vi "Convex Hull 2D (GiftWrap).vi"(0 "Points":sgl[][](array[numeric])=[[0.0, 0.0, 0.0], [10.0, 0.0, 0.0], [10.0, 10.0, 0.0], [0.0, 10.0, 0.0], [50.0, 50.0, 0.0], [60.0, 50.0, 0.0], [60.0, 60.0, 0.0], [50.0, 60.0, 0.0]]) -> (1 "Convex Hull lines":T1[](array[typedef]), 2 "Convex Hull vertices":sgl[][](array[numeric]))   [LabVIEW 2016]
uses:
  Typedefs/Edge, indexed.ctl
  Subroutines/Cross product 3D.vi
  Subroutines/Unit vector.vi
panel:
  # "PN 17/03/2015"
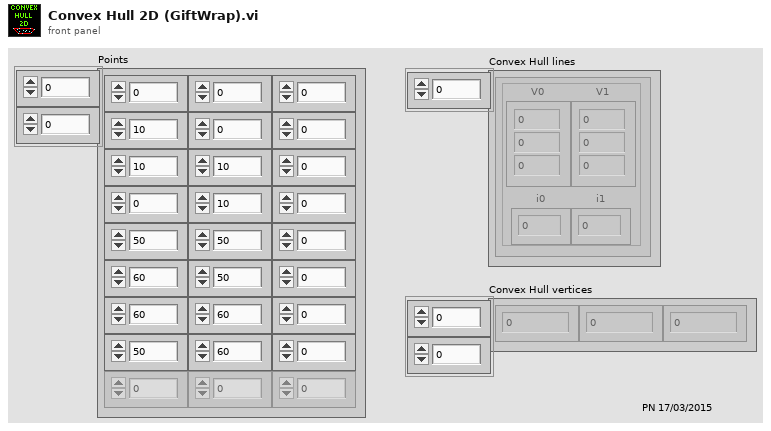
[diagram p1: front panel]
types:
  T1 = typedef "Edge, indexed.ctl" = cluster{"V0":sgl[], "V1":sgl[], "i0":i32, "i1":i32}
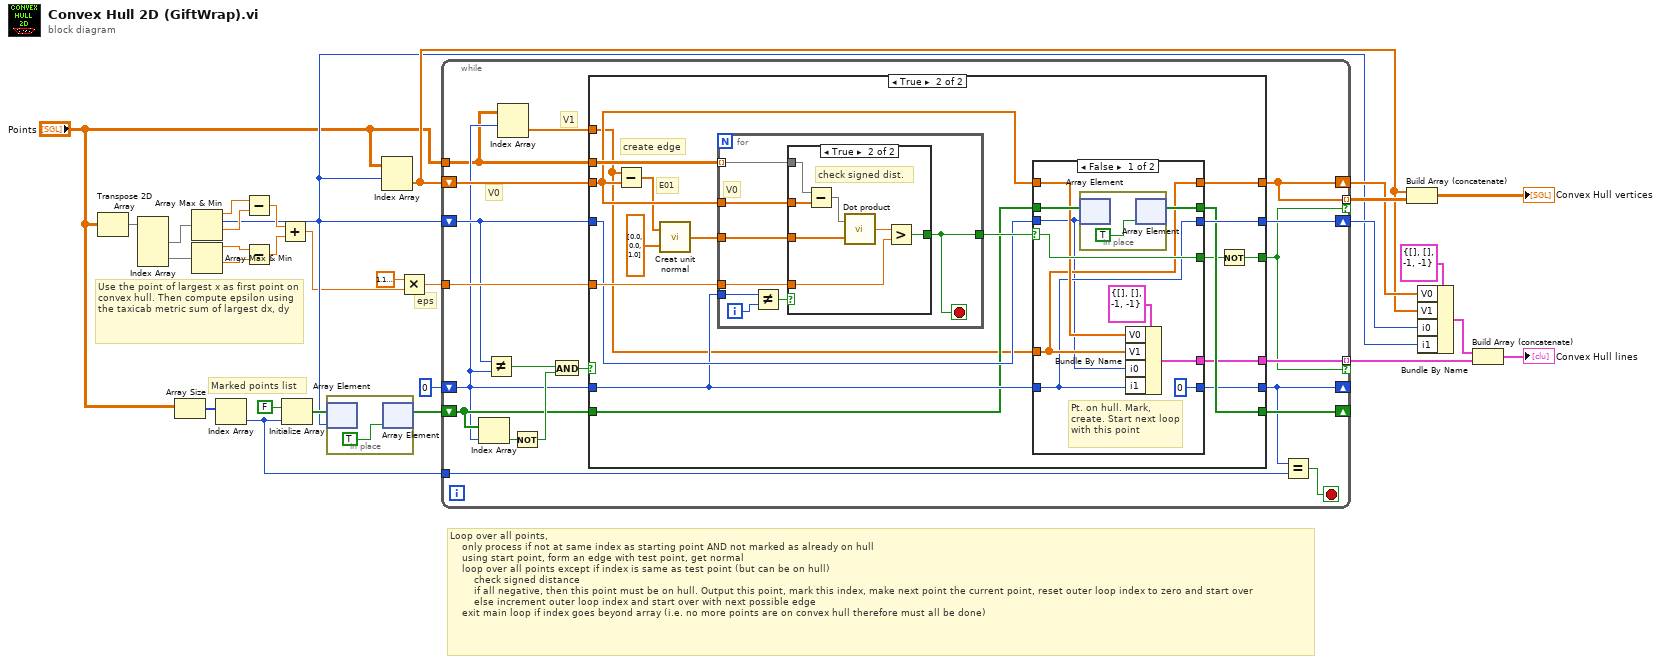
[diagram p0: block diagram]
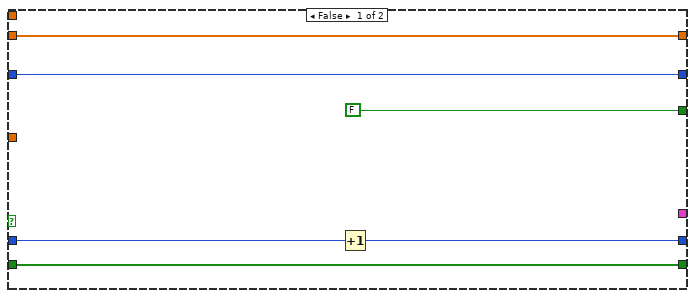
[diagram p2: hidden frame]
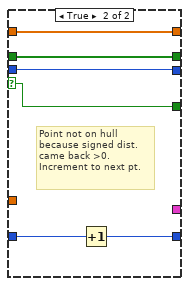
[diagram p3: hidden frame]
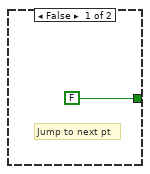
[diagram p4: hidden frame]
diagram:
  # "Use the point of largest x as first point on convex hull. Then compute epsilon using the taxicab metric sum of largest dx, dy"
  # "Loop over all points,\n    only process if not at same index as starting point AND not marked as already on hull\n    using start point, form an edge with test point, get normal\n    loop over all points except if index is same as test point (but can be on hull)\n        check signed distance\n        if all negative, then this point must be on hull. Output this point, mark this index, make next point the current point, reset outer loop index to zero and start over\n        else increment outer loop index and start over with next possible edge\n    exit main loop if index goes beyond array (i.e. no more points are on convex hull therefore must all be done)"
  # "Marked points list"
  # "eps"
  n1 = Transpose 2D Array(2D array="Points") -> (transposed array=w12:sgl[][])
  n2 = Index Array(array=w12) -> (element #1=w11:sgl[], element #2=w10:sgl[])  [unwired: 4 in]
  n3 = Array Size(array="Points") -> (size(s)=w26:i32[])
  n4 = Array Max & Min(array=w11) -> (max value=w9:sgl, max index (indices)=w3:i32, min value=w8:sgl)  [unwired: 1 out]
  n5 = Array Max & Min(array=w10) -> (max value=w7:sgl, min value=w6:sgl)  [unwired: 2 out]
  n6 = Index Array(array=w26) -> (element=w24:i32)  [unwired: 1 in]
  n7 = Subtract(x=w9, y=w8) -> (x-y=w5:sgl)
  n8 = Subtract(x=w7, y=w6) -> (x-y=w4:sgl)
  n9 = Add(x=w5, y=w4) -> (x+y=w2:sgl)
  n10 = Initialize Array(FALSE, w24) -> (w15:bool[])
  n11 = in-place {
    n12 = in-place-array #1(w15, w3) -> ()  [unwired: 1 out]
    n13 = in-place-array #1(TRUE) -> (w14:bool[])  [unwired: 1 out]
  }
  n14 = Index Array(array="Points", index (row)=w3) -> (element=w17:sgl[])  [unwired: 1 in]
  n15 = Multiply(x=sgl 1.1920929e-07, y=w2) -> (x*y=w28:sgl)
  n16 = while {
    shift-right: [w33] -> w18
    shift-left: w17 -> [w49]
    tunnel: w28 -> [w48]
    shift-right: [w46] -> w13
    shift-left: w3 -> [w47]
    shift-right: [w45] -> _
    shift-left: w14 -> [w39]
    tunnel: [w41] -> w20 mode=indexing if=w32
    shift-right: [w35] -> _
    shift-left: 0 -> [w38]
    tunnel: w24 -> [w34]
    tunnel: [w33] -> w23 mode=indexing if=w32
    tunnel: "Points" -> [w31]
    stop <- w36 stop-if-true
    # "V1"
    # "V0"
    n17 = Index Array(array=w39, index=w38) -> (element=w37:bool)
    n18 = Not Equal?(x=w47, y=w38) -> (x != y?=w44:bool)
    n19 = Index Array(array=w31, index (row)=w38) -> (element=w40:sgl[])  [unwired: 1 in]
    n20 = Not(x=w37) -> (.not. x?=w43:bool)
    n21 = And(x=w44, y=w43) -> (x .and. y?=w42:bool)
    n22 = case shown="True" w42 {
      tunnel: w38 -> [w51 w68]
      tunnel: w40 -> [_ w56]
      tunnel: w49 -> [w55 w63]
      tunnel: w48 -> [_ w72]
      tunnel: w31 -> [_ w64]
      tunnel: w47 -> [w54 w70]
      tunnel: [w54 w69] -> w46
      tunnel: [w55 w67] -> w33
      tunnel: w39 -> [w53 w66]
      tunnel: [w53 w65] -> w45
      tunnel: [_ w62] -> w41
      tunnel: [FALSE w60] -> w32
      tunnel: [w50 w57] -> w35
      frame False {
        n23 = Increment(x=w51) -> (x+1=w50:i32)
      }
      frame True {
        # "E01"
        # "create edge"
        n24 = Subtract(x=w56, y=w63) -> (x-y=w58:sgl[])
        n25 = call "Creat unit normal.vi"("E2"=sgl[] [0.0, 0.0, 1.0] ("B"), "E1"=w58) -> ("n^ = (E1 x E2) / ||E1 x E2||"=w59:sgl[])
        n26 = for {
          tunnel: w59 -> [w95]
          tunnel: w64 -> [w94] mode=indexing
          tunnel: w68 -> [w97]
          tunnel: w63 -> [w93]
          tunnel: w72 -> [w92]
          tunnel: [w91] -> w71
          i -> [w98]
          stop <- w91 stop-if-true
          # "V0"
          n27 = Not Equal?(x=w97, y=w98) -> (x != y?=w96:bool)
          n28 = case shown="True" w96 {
            tunnel: w95 -> [_ w106]
            tunnel: w94 -> [_ w105]
            tunnel: w93 -> [_ w104]
            tunnel: [FALSE w100] -> w91
            tunnel: w92 -> [_ w101]
            frame False {
              # "Jump to next pt"
            }
            frame True {
              # "check signed dist."
              n29 = Subtract(x=w105, y=w104) -> (x-y=w103:sgl[])
              n30 = call "Dot product.vi"("B"=w106, "A"=w103) -> ("A . B"=w102:sgl)
              n31 = Greater?(x=w102, y=w101) -> (0:w100:bool)
            }
          }
        }
        n32 = case shown="False" w71 {
          selector: w71 -> [w79 w87]
          tunnel: w70 -> [w74 w89]
          tunnel: [w75 w89] -> w69
          tunnel: w68 -> [w75 w86]
          tunnel: w56 -> [w76 _]
          tunnel: [w76 w90] -> w67
          tunnel: w66 -> [w83 w88]
          tunnel: w63 -> [w78 w90]
          tunnel: [w82 w88] -> w65
          tunnel: [w80 _] -> w62
          tunnel: [w79 w87] -> w61
          tunnel: [0 w85] -> w57
          frame False {
            # "Pt. on hull. Mark, create. Start next loop with this point"
            n33 = in-place {
              n34 = in-place-array #2(w83, w74) -> ()  [unwired: 1 out]
              n35 = in-place-array #2(TRUE) -> (w82:bool[])  [unwired: 1 out]
            }
            n36 = Bundle By Name(cluster=T1 {"V0"=[], "V1"=[], "i0"=-1, "i1"=-1} ("Edge, indexed"), "V0"=w78, "V1"=w76, "i0"=w74, "i1"=w75) -> (w80:T1)
          }
          frame True {
            # "Point not on hull because signed dist. came back >0.\nIncrement to next pt."
            n37 = Increment(x=w86) -> (x+1=w85:i32)
          }
        }
        n38 = Not(x=w61) -> (.not. x?=w60:bool)
      }
    }
    n39 = Equal?(x=w35, y=w34) -> (x = y?=w36:bool)
  }
  n40 = Build Array (concatenate)(w17, w23) -> (→"Convex Hull vertices":sgl[][])
  n41 = Bundle By Name(cluster=T1 {"V0"=[], "V1"=[], "i0"=-1, "i1"=-1} ("Edge, indexed"), "V0"=w18, "V1"=w17, "i0"=w13, "i1"=w3) -> (w16:T1)
  n42 = Build Array (concatenate)(w16, w20) -> (→"Convex Hull lines":T1[])
